vi "HMI Logic.vi"(7 "Device":T5, 8 "error in (no error)":errorcluster, 9 "Expo":dbl, 10 "HMI":T1={"button info"={"button 1"=FALSE, "button 2"=FALSE, "button 3"=FALSE, "button 4"=FALSE, "button 5"=FALSE, "button 6"=FALSE, "button 7"=FALSE, "button 8"=FALSE, "button 9"=FALSE, "button 10"=FALSE, "button 11"=FALSE, "button 12"=FALSE, "button 13"=FALSE, "button 14"=FALSE, "button 15"=FALSE, "button 16"=FALSE, "button 17"=FALSE, "button 18"=FALSE, "button 19"=FALSE, "button 20"=FALSE, "button 21"=FALSE, "button 22"=FALSE, "button 23"=FALSE, "button 24"=FALSE, "button 25"=FALSE, "button 26"=FALSE, "button 27"=FALSE, "button 28"=FALSE, "button 29"=FALSE, "button 30"=FALSE, "button 31"=FALSE, "button 32"=FALSE}, "direction info"={"pov 1"=-1, "pov 2"=-1, "pov 3"=-1, "pov 4"=-1}, "axis info"={"X axis"=3832, "Y axis"=898, "Z axis"=0, "X axis rotation"=-443, "Y axis rotation"=465, "Z axis rotation"=0, "U axis"=0, "V axis"=0}}, 11 "Steering Frame in":T4) -> (0 "error out":errorcluster, 3 "Steering Frame out":T4)   [LabVIEW 2012]
uses:
  <vilib>/robotics/Steering/Class Type Definitions/Mecanum Steering Frame.ctl
  <vilib>/robotics/Steering/Mecanum Steering Frame/NI_Robotics_Mecanum Steering Frame.lvclass
  <vilib>/robotics/Steering/Class Type Definitions/Differential Steering Frame.ctl
  <vilib>/robotics/Steering/Differential Steering Frame/NI_Robotics_Differential Steering Frame.lvclass
  <vilib>/robotics/Steering/Class Type Definitions/NI_Robotics_Steering Class Types.lvlib
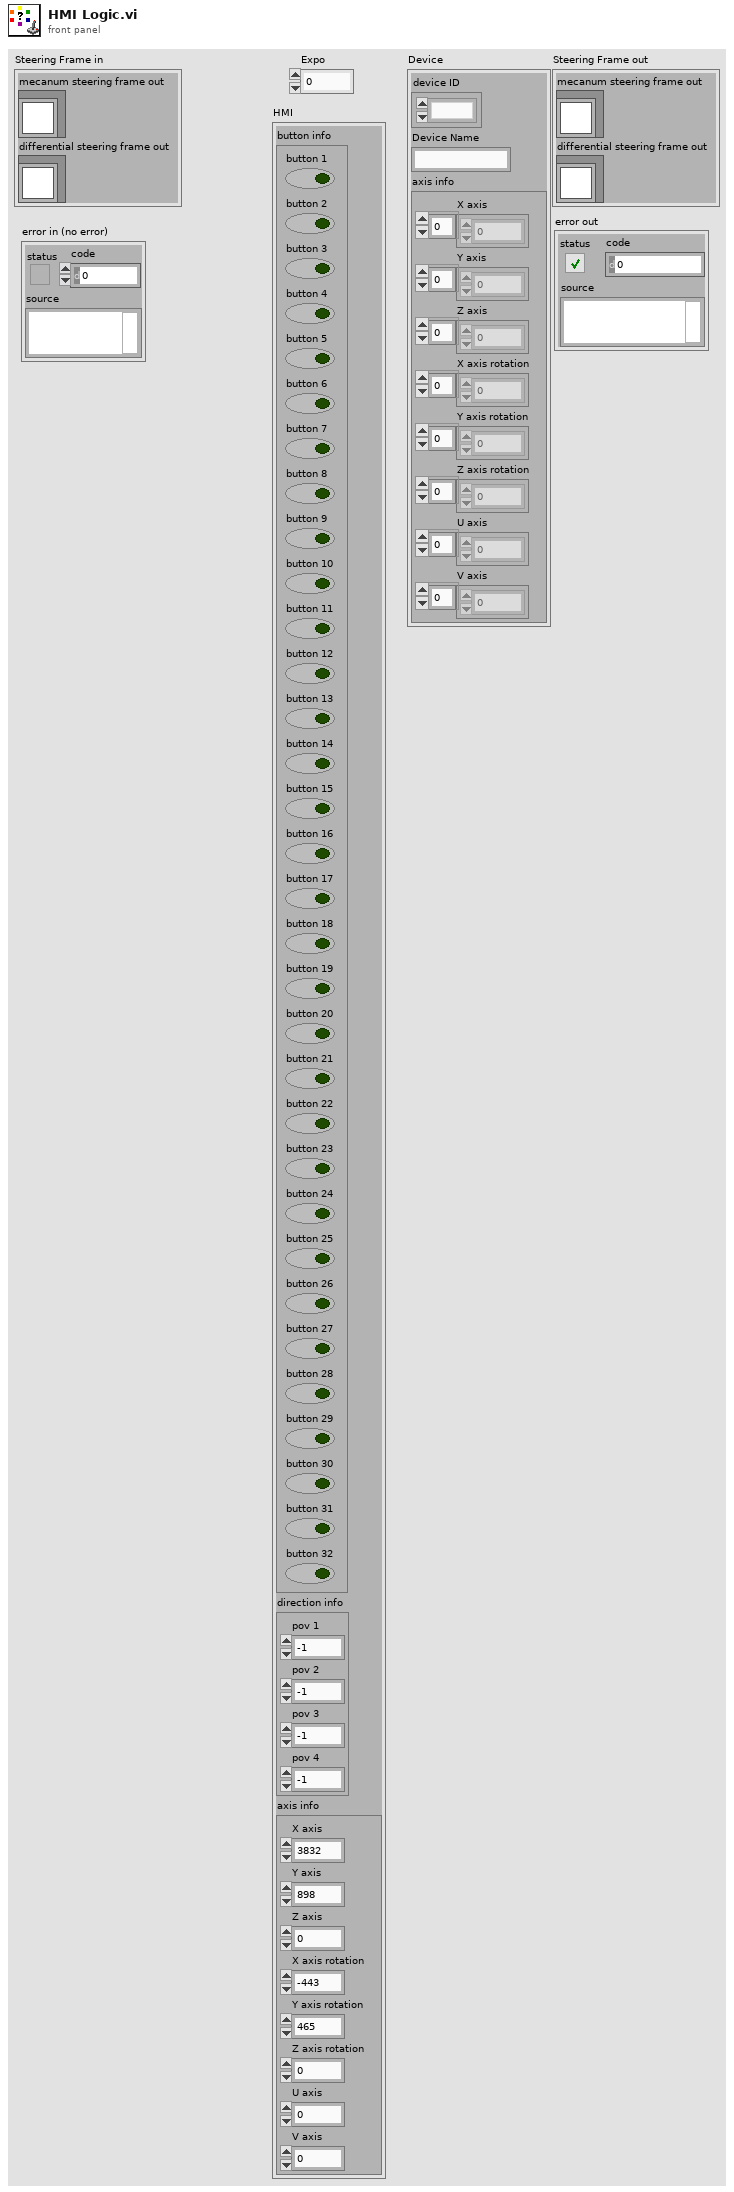
[diagram p1: front panel]
types:
  T1 = cluster{"button info":cluster{"button 1":bool, "button 2":bool, "button 3":bool, "button 4":bool, "button 5":bool, "button 6":bool, "button 7":bool, "button 8":bool, "button 9":bool, "button 10":bool, "button 11":bool, "button 12":bool, "button 13":bool, "button 14":bool, "button 15":bool, "button 16":bool, "button 17":bool, "button 18":bool, "button 19":bool, "button 20":bool, "button 21":bool, "button 22":bool, "button 23":bool, "button 24":bool, "button 25":bool, "button 26":bool, "button 27":bool, "button 28":bool, "button 29":bool, "button 30":bool, "button 31":bool, "button 32":bool}, "direction info":cluster{"pov 1":i32, "pov 2":i32, "pov 3":i32, "pov 4":i32}, "axis info":cluster{"X axis":i32, "Y axis":i32, "Z axis":i32, "X axis rotation":i32, "Y axis rotation":i32, "Z axis rotation":i32, "U axis":i32, "V axis":i32}}
  T2 = typedef "NI_Robotics_Steering Class Types.lvlib/Mecanum Steering Frame.ctl" = refnum<class "NI_Robotics_Mecanum Steering Frame.lvclass">
  T3 = typedef "NI_Robotics_Steering Class Types.lvlib/Differential Steering Frame.ctl" = refnum<class "NI_Robotics_Differential Steering Frame.lvclass">
  T4 = cluster{"mecanum steering frame out":T2, "differential steering frame out":T3}
  T5 = cluster{"device ID":refnum<k1>, "Device Name":string, "axis info":cluster{"X axis":dbl[], "Y axis":dbl[], "Z axis":dbl[], "X axis rotation":dbl[], "Y axis rotation":dbl[], "Z axis rotation":dbl[], "U axis":dbl[], "V axis":dbl[]}}
  T6 = cluster{"button 1":bool, "button 2":bool, "button 3":bool, "button 4":bool, "button 5":bool, "button 6":bool, "button 7":bool, "button 8":bool, "button 9":bool, "button 10":bool, "button 11":bool, "button 12":bool, "button 13":bool, "button 14":bool, "button 15":bool, "button 16":bool, "button 17":bool, "button 18":bool, "button 19":bool, "button 20":bool, "button 21":bool, "button 22":bool, "button 23":bool, "button 24":bool, "button 25":bool, "button 26":bool, "button 27":bool, "button 28":bool, "button 29":bool, "button 30":bool, "button 31":bool, "button 32":bool}
  T7 = cluster{"pov 1":i32, "pov 2":i32, "pov 3":i32, "pov 4":i32}
  T8 = cluster{"X axis":i32, "Y axis":i32, "Z axis":i32, "X axis rotation":i32, "Y axis rotation":i32, "Z axis rotation":i32, "U axis":i32, "V axis":i32}
  T9 = cluster{"X axis":dbl, "Y axis":dbl, "Z axis":dbl, "X axis rotation":dbl, "Y axis rotation":dbl, "Z axis rotation":dbl, "U axis":dbl, "V axis":dbl}
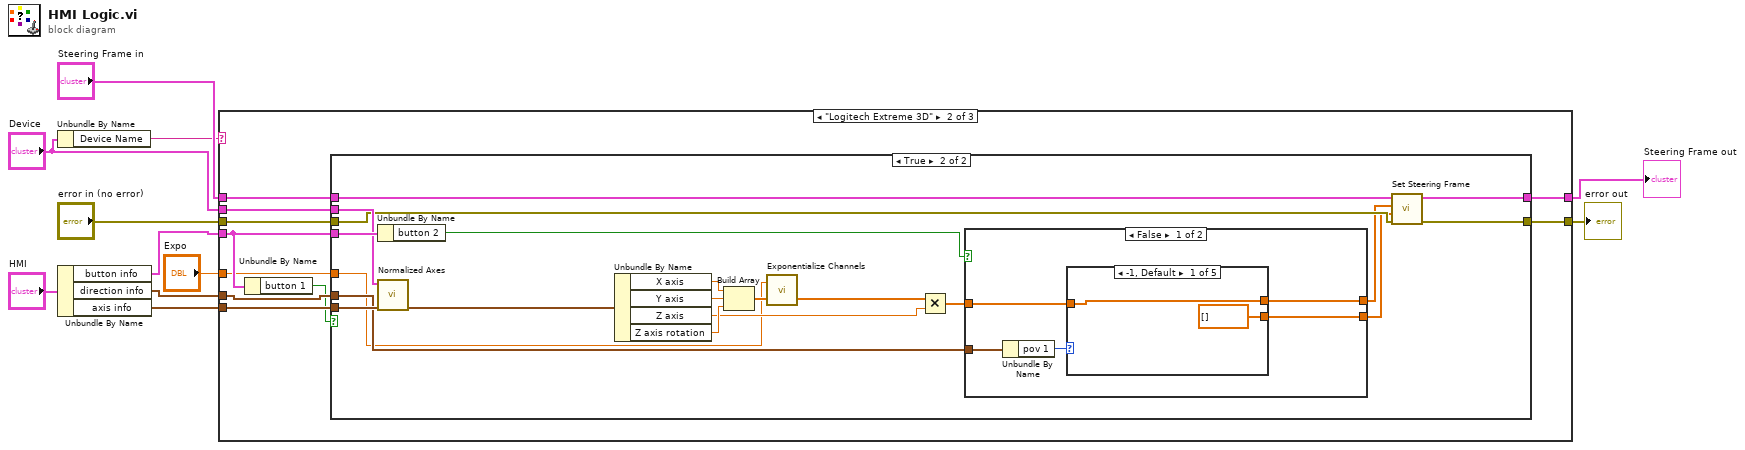
[diagram p0: block diagram]
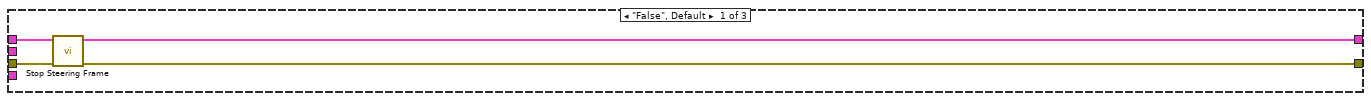
[diagram p2: hidden frame]
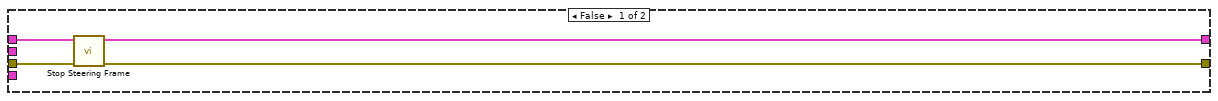
[diagram p3: hidden frame]
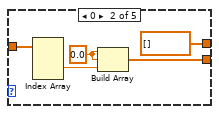
[diagram p4: hidden frame]
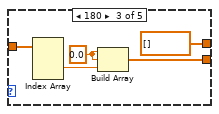
[diagram p5: hidden frame]
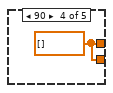
[diagram p6: hidden frame]
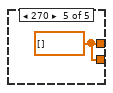
[diagram p7: hidden frame]
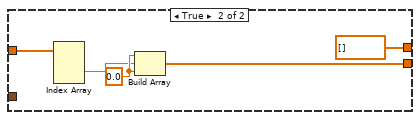
[diagram p8: hidden frame]
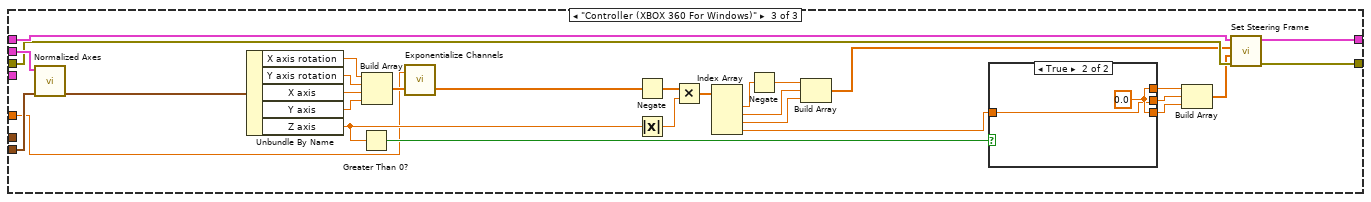
[diagram p9: hidden frame]
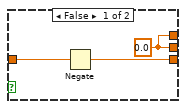
[diagram p10: hidden frame]
diagram:
  n1 = Unbundle By Name("Device") -> ("Device Name"=w7:string)
  n2 = Unbundle By Name("HMI") -> ("button info"=w3:T6, "direction info"=w2:T7, "axis info"=w1:T8)
  n3 = case shown="\"Logitech Extreme 3D\"" w7 {
    tunnel: w3 -> [_ w21 _]
    tunnel: w1 -> [_ w25 w102]
    tunnel: w2 -> [_ w23 _]
    tunnel: "Device" -> [_ w24 w101]
    tunnel: "Steering Frame in" -> [w14 w22 w100]
    tunnel: "error in (no error)" -> [w15 w19 w99]
    tunnel: [w12 w18 w98] -> w5
    tunnel: [w13 w17 w97] -> w6
    tunnel: "Expo" -> [_ w16 w74]
    frame "False", Default {
      n4 = call "Stop Steering Frame.vi"("error in (no error)"=w15, "Steering Frame in"=w14) -> ("error out"=w12:errorcluster, "Steering Frame out"=w13:T4)  [unwired: 8 in]
    }
    frame "Logitech Extreme 3D" {
      n5 = Unbundle By Name(w21) -> ("button 1"=w20:bool)
      n6 = case shown="True" w20 {
        tunnel: w25 -> [_ w45]
        tunnel: w24 -> [_ w37]
        tunnel: w23 -> [_ w41]
        tunnel: w21 -> [_ w43]
        tunnel: w22 -> [w26 w33]
        tunnel: [w27 w34] -> w17
        tunnel: w19 -> [w29 w36]
        tunnel: [w28 w35] -> w18
        tunnel: w16 -> [_ w30]
        frame False {
          n7 = call "Stop Steering Frame.vi"("error in (no error)"=w29, "Steering Frame in"=w26) -> ("error out"=w28:errorcluster, "Steering Frame out"=w27:T4)  [unwired: 8 in]
        }
        frame True {
          n8 = Unbundle By Name(w43) -> ("button 2"=w42:bool)
          n9 = call "Normalized Axes.vi"("axis in"=w45, "Device in"=w37) -> ("axis out"=w47:T9)  [unwired: 8 in, 1 out]
          n10 = Unbundle By Name(w47) -> ("X axis"=w48:dbl, "Y axis"=w49:dbl, "Z axis"=w40:dbl, "Z axis rotation"=w44:dbl)
          n11 = Build Array(w48, w49, w44) -> (w46:dbl[])
          n12 = call "Exponentialize Channels.vi"("Channels in"=w46, "Expo"=w30) -> ("Channels out"=w39:dbl[])  [unwired: 1 in]
          n13 = Multiply(x=w39, y=w40) -> (x*y=w38:dbl[])
          n14 = case shown="False" w42 {
            tunnel: [w54 dbl[] []] -> w32
            tunnel: [w53 w70] -> w31
            tunnel: w41 -> [w52 _]
            tunnel: w38 -> [w50 w72]
            frame False {
              n15 = Unbundle By Name(w52) -> ("pov 1"=w51:i32)
              n16 = case shown="-1, Default" w51 {
                tunnel: w50 -> [w56 w61 w66 _ _]
                tunnel: [w56 dbl[] [] dbl[] [] w67 w68] -> w54
                tunnel: [dbl[] [] w57 w62 w67 w68] -> w53
                frame -1, Default {
                }
                frame 0 {
                  w59 = 0.0 ("element")
                  n17 = Index Array(array=w61) -> (element #2=w60:dbl)  [unwired: 3 in, 2 out]
                  n18 = Build Array(w59, w59, w60) -> (w57:dbl[])
                }
                frame 180 {
                  w64 = 0.0 ("element")
                  n19 = Index Array(array=w66) -> (element #2=w65:dbl)  [unwired: 3 in, 2 out]
                  n20 = Build Array(w64, w64, w65) -> (w62:dbl[])
                }
                frame 90 {
                  w67 = dbl[] []
                }
                frame 270 {
                  w68 = dbl[] []
                }
              }
            }
            frame True {
              w71 = 0.0 ("element")
              n21 = Index Array(array=w72) -> (element #2=w69:dbl)  [unwired: 3 in, 2 out]
              n22 = Build Array(w71, w69, w71) -> (w70:dbl[])
            }
          }
          n23 = call "Set Steering Frame.vi"("error in (no error)"=w36, "differential frame velocity"=w31, "mecanum frame velocity"=w32, "Steering Frame in"=w33) -> ("error out"=w35:errorcluster, "Steering Frame out"=w34:T4)  [unwired: 6 in]
        }
      }
    }
    frame "Controller (XBOX 360 For Windows)" {
      n24 = call "Normalized Axes.vi"("axis in"=w102, "Device in"=w101) -> ("axis out"=w96:T9)  [unwired: 8 in, 1 out]
      n25 = Unbundle By Name(w96) -> ("X axis rotation"=w92:dbl, "Y axis rotation"=w91:dbl, "X axis"=w90:dbl, "Y axis"=w89:dbl, "Z axis"=w84:dbl)
      n26 = Greater Than 0?(x=w84) -> (x > 0?=w83:bool)
      n27 = Build Array(w92, w91, w90, w89) -> (w88:dbl[])
      n28 = call "Exponentialize Channels.vi"("Channels in"=w88, "Expo"=w74) -> ("Channels out"=w95:dbl[])  [unwired: 1 in]
      n29 = Negate(x=w95) -> (-x=w78:dbl[])
      n30 = Absolute Value(x=w84) -> (abs(x)=w85:dbl)
      n31 = Multiply(x=w78, y=w85) -> (x*y=w94:dbl[])
      n32 = Index Array(array=w94) -> (element #1=w87:dbl, element #2=w76:dbl, element #3=w77:dbl, element #4=w82:dbl)  [unwired: 4 in]
      n33 = Negate(x=w87) -> (-x=w75:dbl)
      n34 = Build Array(w75, w76, w77) -> (w86:dbl[])
      n35 = case shown="True" w83 {
        tunnel: w82 -> [w105 w106]
        tunnel: [w104 w107] -> w81
        tunnel: [w104 w106] -> w80
        tunnel: [w103 w107] -> w79
        frame False {
          w104 = 0.0 ("element")
          n36 = Negate(x=w105) -> (-x=w103:dbl)
        }
        frame True {
          w107 = 0.0 ("element")
        }
      }
      n37 = Build Array(w81, w80, w79) -> (w93:dbl[])
      n38 = call "Set Steering Frame.vi"("error in (no error)"=w99, "differential frame velocity"=w93, "mecanum frame velocity"=w86, "Steering Frame in"=w100) -> ("error out"=w98:errorcluster, "Steering Frame out"=w97:T4)  [unwired: 6 in]
    }
  }
  "Steering Frame out" <- w6
  "error out" <- w5
